vi "Init Res Table.vi"(7 "Groups":u8[](array[numeric]), 11 "Channels":string[](array[string])) -> ()   [LabVIEW 2020]
uses:
  <vilib>/Utility/miscctls.llb/LVRowAndColumnTypeDef.ctl
  support/REF Single  Name to ref convert.vi
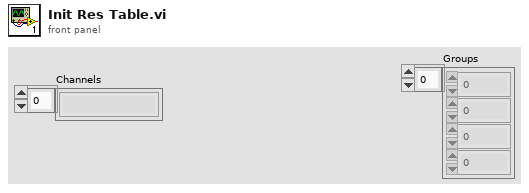
[diagram p1: front panel]
types:
  T1 = typedef "LVRowAndColumnTypeDef.ctl" = cluster{"Row":i32, "Column":i32}
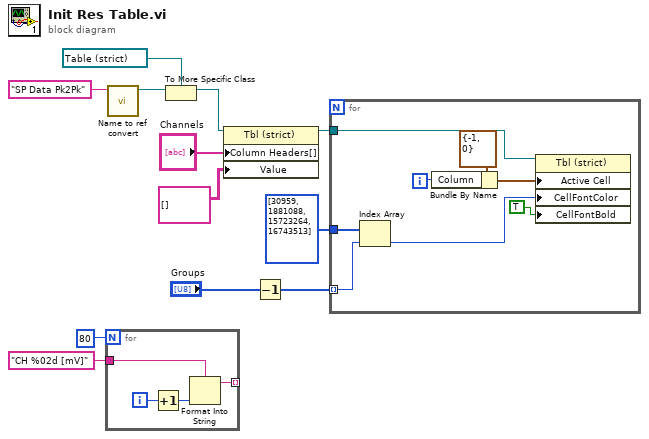
[diagram p0: block diagram]
diagram:
  n1 = for {
    N: 80 -> [_]
    tunnel: [w14] -> _ mode=indexing
    tunnel: "CH %02d [mV]" ("format string") -> [w13]
    i -> [w16]
    n2 = Increment(x=w16) -> (x+1=w15:i32)
    n3 = Format Into String(format string=w13, w15) -> (resulting string=w14:string)  [unwired: 2 in, 1 out]
  }
  n4 = call-poly "Name to ref convert.vi"("name"="SP Data Pk2Pk") -> ("First REF"=w6:refnum<vi>)  [unwired: 10 in]
  n5 = To More Specific Class(target class=refnum<vi> refnum ("Limit Table"), reference=w6) -> (specific class reference=w9:refnum<vi>)  [unwired: 1 in, 1 out]
  n6 = property on="Property Node" class="Tbl (strict)"(reference=w9, "Column Headers[]"="Channels", "Value"=string[][] []) -> (reference out=w4:refnum<vi>)  [unwired: 1 in, 1 out]
  n7 = Decrement(x="Groups") -> (x-1=w1:u8[])
  n8 = for {
    tunnel: w4 -> [w24]
    tunnel: w1 -> [w22] mode=indexing
    tunnel: u32[] [30959, 1881088, 15723264, 16743513] -> [w23]
    i -> [w18]
    n9 = Index Array(array=w23, index=w22) -> (element=w21:u32)
    n10 = Bundle By Name(cluster=T1 {"Row"=-1, "Column"=0} ("Active Cell:Active Cell"), "Column"=w18) -> (w19:T1)
    n11 = property on="Property Node" class="Tbl (strict)"(reference=w24, "Active Cell"=w19, "CellFontColor"=w21, "CellFontBold"=TRUE ("Active Cell:Cell Font:Bold")) -> ()  [unwired: 1 in, 2 out]
  }
